vi "Eject CD.vi"(0 "Drive to Eject (E:\\)":path=path "E:/") -> ()   [LabVIEW 2011]
doc: "Uses the Microsoft Multimedia ActiveX control (MCI Version 6) to eject a CD on the input drive. If the CD drive supports it, the tray can also be closed again by calling this VI. Requires the MM control to be installed and registered."
panel:
  out "CanEject":bool
  in  "MCI.Imci":refnum<k7>(container)
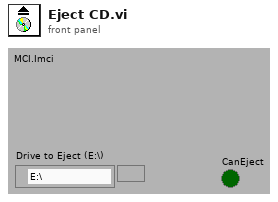
[diagram p1: front panel]
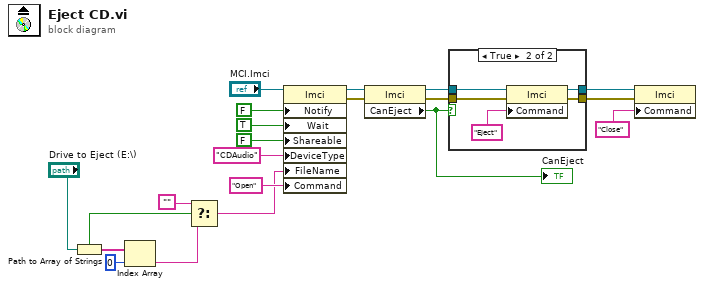
[diagram p0: block diagram]
diagram:
  n1 = Path to Array of Strings(0:"Drive to Eject (E:\\)") -> (1:w6:bool, 2:w5:string[])
  n2 = Index Array(array=w5, index=0 ("Index")) -> (element=w2:string)
  n3 = Select(t="", s=w6, f=w2) -> (s? t:f=w1:string)
  n4 = property class="Imci"(reference="MCI.Imci", "Notify"=FALSE, "Wait"=TRUE, "Shareable"=FALSE, "DeviceType"="CDAudio", "FileName"=w1, "Command"="Open") -> (reference out=w13:refnum<k7>, error out=w10:errorcluster)  [unwired: 1 in]
  n5 = property class="Imci"(reference=w13, error in=w10) -> (reference out=w12:refnum<k7>, error out=w11:errorcluster, "CanEject"=w8:bool)
  "CanEject" <- w8
  n6 = case shown="True" w8 {
    tunnel: [w23 w28] -> w15
    tunnel: [w22 w27] -> w14
    tunnel: w12 -> [w23 w25]
    tunnel: w11 -> [w22 w24]
    frame False {
    }
    frame True {
      n7 = property class="Imci"(reference=w25, error in=w24, "Command"="Eject") -> (reference out=w28:refnum<k7>, error out=w27:errorcluster)
    }
  }
  n8 = property class="Imci"(reference=w15, error in=w14, "Command"="Close") -> ()  [unwired: 2 out]
